vi "Thor.GetTandH.vi"(8 "error in (no error)":errorcluster, 10 "Thorlabs type":enum16{"A", "B"}(ring), 11 "Thorlabs handle out":refnum<visa-resource-name>) -> (0 "error out":errorcluster, 2 "Humidity":dbl, 3 "Temperature":dbl)   [LabVIEW 2019, in "TEMPerHUM.lvlib"]
uses:
  TEMPerHUM.lvlib
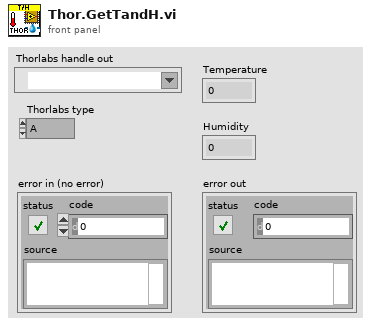
[diagram p1: front panel]
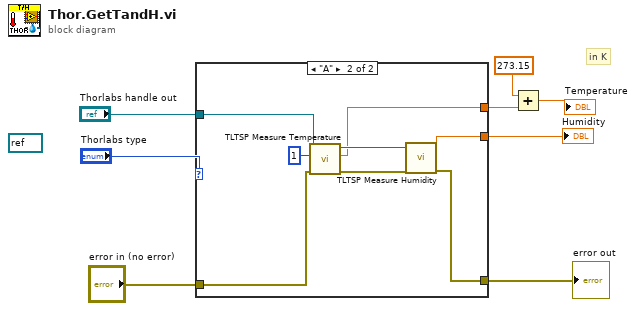
[diagram p0: block diagram]
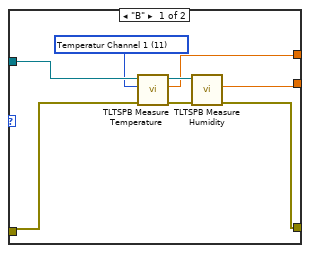
[diagram p2: hidden frame]
diagram:
  (unwired) refnum<visa-resource-name> refnum ("instrument handle out")
  # "in K"
  n1 = case shown="\"A\"" "Thorlabs type" {
    tunnel: [w12 w22] -> w3
    tunnel: [w15 w21] -> w8
    tunnel: "error in (no error)" -> [w11 w20]
    tunnel: [w9 w18] -> w6
    tunnel: "Thorlabs handle out" -> [w16 w17]
    frame "B" {
      w14 = u16 11 items=["Temperatur Channel 1"=11, "Temperatur Channel 2"=12, "Temperatur Channel 3"=13] ("Channel (Temperatur Channel 1)")
      n2 = call <instrlib>:"TLTSPB Measure Temperature.vi"("error in (no error)"=w11, "Channel (Temperatur Channel 1)"=w14, "instrument handle"=w16) -> ("error out"=w10:errorcluster, "Temperature"=w12:dbl, "instrument handle out"=w13:refnum<visa-resource-name>)  [unwired: 6 in]
      n3 = call <instrlib>:"TLTSPB Measure Humidity.vi"("error in (no error)"=w10, "instrument handle"=w13) -> ("error out"=w9:errorcluster, "Humidity"=w15:dbl)  [unwired: 7 in, 1 out]
    }
    frame "A" {
      n4 = call <instrlib>:"TLTSP Measure Temperature.vi"("error in (no error)"=w20, "Channel (1)"=u16 1, "instrument handle"=w17) -> ("error out"=w19:errorcluster, "Temperature"=w22:dbl, "instrument handle out"=w24:refnum<visa-resource-name>)  [unwired: 6 in]
      n5 = call <instrlib>:"TLTSP Measure Humidity.vi"("error in (no error)"=w19, "instrument handle"=w24) -> ("error out"=w18:errorcluster, "Humidity"=w21:dbl)  [unwired: 7 in, 1 out]
    }
  }
  "Humidity" <- w8
  "error out" <- w6
  n6 = Add(x=273.15, y=w3) -> (x+y=→"Temperature":dbl)
